vi "Set Chamber Pressure Valve.vi"(8 "error in (no error)":errorcluster, 10 "State":T1, 11 "Process Settings in":refnum<class "Process Settings.lvclass">) -> (0 "error out":errorcluster, 3 "Process Settings out":refnum<class "Process Settings.lvclass">)   [LabVIEW 2017, in "Saturation.lvclass"]
uses:
  Saturation.lvclass
  Process Settings/Process Settings.lvclass
  Type Defs/Valve State.ctl
  Hardware Settings/Type Defs/Hardware Types.ctl
  Process Settings/Type Defs/Item.ctl
  Process Settings/Process Settings.lvclass/Process Settings.ctl
  Process Settings/Accessors/Read Hardware Settings.vi
  Hardware Settings/Hardware Settings.lvclass
  Hardware Settings/Hardware Types/Generic/Generic Hardware.lvclass
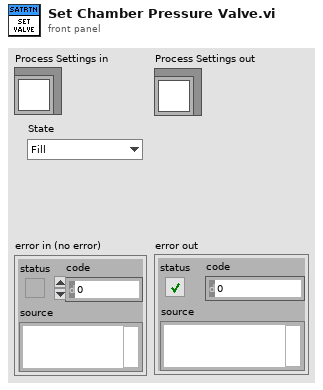
[diagram p1: front panel]
types:
  T1 = typedef "Saturation.lvclass/Valve State.ctl" = enum16{"Fill", "Saturate", "Exhaust"}
  T2 = typedef "Process Settings.lvclass/Item.ctl" = enum16{"", "sheet temperature setpoint", "sheet heating time", "temp element setpoint", "chamber pressure setpoint", "saturation time", "chamber pressure valve setpoint"}
  T3 = typedef "Hardware Settings.lvclass/Hardware Types.ctl" = enum16{"Tank Chamber Pressure and Temperature", "Tank Valve Controls", "Motor On/Off and Direction Control", "Limit Switches", "IR Temperature", "Pneumatic Cylinder Actuation", "Expansion Temperature Setpoint"}
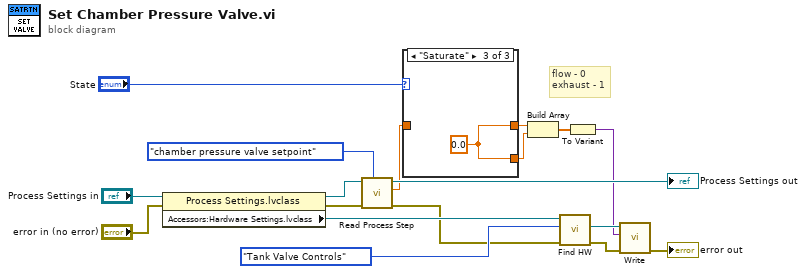
[diagram p0: block diagram]
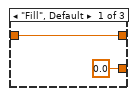
[diagram p2: hidden frame]
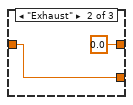
[diagram p3: hidden frame]
diagram:
  # "flow - 0 \nexhaust - 1"
  n1 = property class="Process Settings.lvclass"(reference="Process Settings in", error in="error in (no error)") -> (reference out=w11:refnum<class "Process Settings.lvclass">, error out=w9:errorcluster, "Accessors:Hardware Settings.lvclass"=w12:refnum<class "Hardware Settings.lvclass">)
  n2 = call "Read Process Step.vi"("Item"=Item."chamber pressure valve setpoint", "error in (no error)"=w9, "Process Settings in"=w11) -> ("error out"=w8:errorcluster, "Value"=w3:dbl, "Process Settings out"=→"Process Settings out":refnum<class "Process Settings.lvclass">)  [unwired: 5 in, 1 out]
  n3 = case shown="\"Saturate\"" "State" {
    tunnel: [w20 0.0 ("f") w23] -> w5
    tunnel: w3 -> [w20 w22 _]
    tunnel: [0.0 ("f") w22 w23] -> w2
    frame "Fill", Default {
    }
    frame "Exhaust" {
    }
    frame "Saturate" {
      w23 = 0.0 ("f")
    }
  }
  n4 = Build Array(w5, w2) -> (w4:dbl[])
  n5 = call "Find HW.vi"("error in (no error)"=w8, "HW Item"=Hardware_Types."Tank Valve Controls", "Hardware Settings in"=w12) -> ("error out"=w18:errorcluster, "Selected Hardware Out"=w17:refnum<class "Generic Hardware.lvclass">)  [unwired: 6 in, 1 out]
  n6 = To Variant(anything=w4) -> (Variant=w6:variant)
  n7 = call-dynamic "Write.vi"("error in (no error)"=w18, "Input"=w6, "Generic Hardware in"=w17) -> ("error out"=→"error out":errorcluster)  [unwired: 7 in, 1 out]
